vi "Initialize Daemon.vi"(8 "error in":errorcluster, 9 "Data Model":refnum<class "Device Data Model.lvclass">, 11 "Serial Slave in":refnum<class "Serial Slave.lvclass">) -> (0 "error out":errorcluster, 3 "Serial Slave out":refnum<class "Serial Slave.lvclass">)   [LabVIEW 2021, in "Serial Slave.lvclass"]
doc: "This provides an interface for the slave to launch a protocol daemon."
uses:
  Serial Slave.lvclass
  Serial Daemon.vi
  Network Interface/Serial Interface/Serial Shared Components/Serial Shared Components.lvlib
  Transmission Data Unit/Transmission Data Unit.lvclass
  Network Protocol.lvclass
  Transmission Data Unit/Serial Interface/Serial Data Unit.lvclass
  Network Slave.lvclass
  C:/my_projects/projects/Algorithms/Labview/21/Modbus_v121c/Network Protocol/Network Slave/Network Slave.lvclass
  C:/my_projects/projects/Algorithms/Labview/21/Modbus_v121c/Network Protocol/Network Protocol.lvclass
  C:/my_projects/projects/Algorithms/Labview/21/Modbus_v121c/Network Protocol/Network Slave/Serial/Serial Slave.lvclass
  Data Model/Device Data Model.lvclass
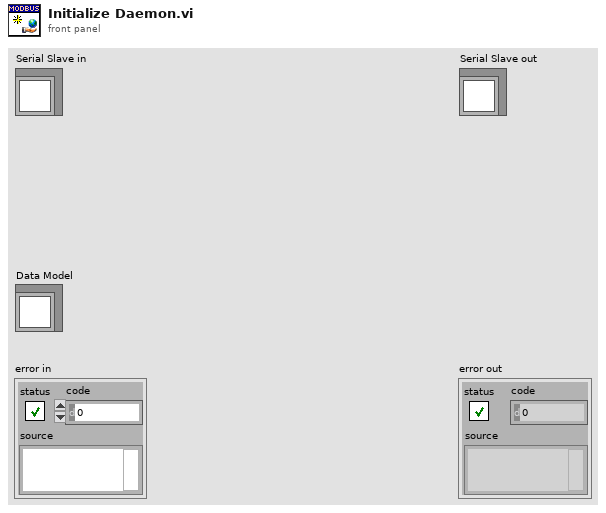
[diagram p1: front panel]
types:
  T1 = enum16{"None", "XON/XOFF", "RTS/CTS", "XON/XOFF & RTS/CTS", "DTR/DSR", "XON/XOFF & DTR/DSR"}
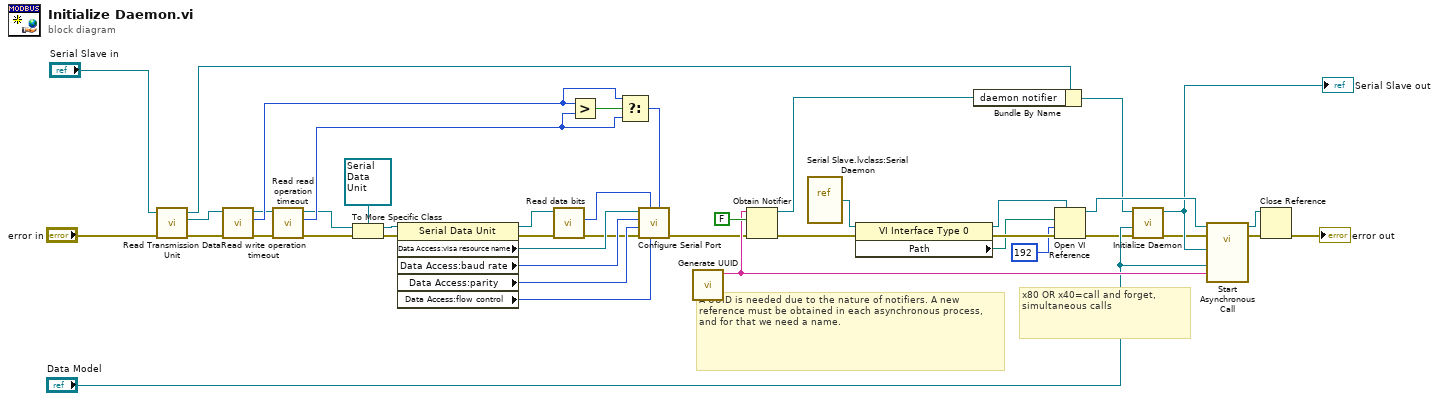
[diagram p0: block diagram]
diagram:
  # "x80 OR x40=call and forget, simultaneous calls"
  # "A UUID is needed due to the nature of notifiers. A new reference must be obtained in each asynchronous process, and for that we need a name."
  n1 = call "Read Transmission Data Unit.vi"("error in (no error)"="error in", "Network Protocol in"="Serial Slave in") -> ("error out"=w13:errorcluster, "Transmission Data Unit"=w5:refnum<class "Transmission Data Unit.lvclass">, "Network Protocol out"=w12:refnum<class "Serial Slave.lvclass">)  [unwired: 7 in]
  n2 = call "Read write operation timeout.vi"("error in (no error)"=w13, "transmission data unit in"=w5) -> ("error out"=w16:errorcluster, "write operation timeout"=w15:i32, "transmission data unit out"=w14:refnum<class "Transmission Data Unit.lvclass">)  [unwired: 7 in]
  n3 = call "Read read operation timeout.vi"("error in (no error)"=w16, "transmission data unit in"=w14) -> ("error out"=w4:errorcluster, "read operation timeout"=w24:i32, "transmission data unit out"=w3:refnum<class "Transmission Data Unit.lvclass">)  [unwired: 7 in]
  n4 = To More Specific Class(target class=refnum<class "Serial Data Unit.lvclass"> refnum ("Serial Data Unit in"), reference=w3, error in=w4) -> (specific class reference=w9:refnum<class "Serial Data Unit.lvclass">, error out=w8:errorcluster)
  n5 = property class="Serial Data Unit"(reference=w9, error in=w8) -> (reference out=w2:refnum<class "Serial Data Unit.lvclass">, error out=w1:errorcluster, "Data Access:visa resource name"=w35:refnum<visa-resource-name>, "Data Access:baud rate"=w33:u32, "Data Access:parity"=w32:enum16{"None", "Odd", "Even", "Mark", "Space"}, "Data Access:flow control"=w31:T1)
  n6 = call-dynamic "Read data bits.vi"("error in (no error)"=w1, "Serial Data Unit in"=w2) -> ("error out"=w7:errorcluster, "data bits"=w34:u16)  [unwired: 7 in, 1 out]
  n7 = Greater?(x=w15, y=w24) -> (0:w25:bool)
  n8 = Select(t=w15, s=w25, f=w24) -> (s? t:f=w23:i32)
  n9 = call "Configure Serial Port.vi"("Timeout"=w23, "Flow Control"=w31, "data bits"=w34, "error in (no error)"=w7, "Parity"=w32, "Baud Rate"=w33, "VISA Refnum in"=w35) -> ("error out"=w30:errorcluster)  [unwired: 4 in]
  n10 = call "Generate UUID.vi"() -> ("UUID"=w37:string)  [unwired: 11 in]
  n11 = Obtain Notifier(name (unnamed)=w37, notification data type=FALSE, error in (no error)=w30) -> (notifier out=w38:refnum<notifier>, error out=w19:errorcluster)  [unwired: 1 in, 1 out]
  n12 = vi-ref "Serial Slave.lvclass:Serial Daemon.vi"() -> (w43:refnum<vi>)
  n13 = property class="VI Interface Type 0"(reference=w43, error in=w19) -> (reference out=w21:refnum<vi>, error out=w42:errorcluster, "Path"=w41:path)
  n14 = Bundle By Name(cluster=w12, "daemon notifier"=w38) -> (w27:refnum<class "Serial Slave.lvclass">)
  n15 = Open VI Reference(type specifier VI Refnum (for type only)=w21, vi path=w41, options=192 ("x .or. y?"), error in (no error)=w42) -> (vi reference=w40:refnum<vi>, error out=w18:errorcluster)  [unwired: 2 in]
  n16 = call-parent "Initialize Daemon.vi"("error in"=w18, "Data Model"="Data Model", "network slave in"=w27) -> ("error out"=w17:errorcluster, "network slave out"=w28:refnum<class "Serial Slave.lvclass">)  [unwired: 7 in]
  "Serial Slave out" <- w28
  n17 = call-by-ref "Start Asynchronous Call"(reference=w40, error in=w17, "UUID"=w37, "Data Model"="Data Model", "serial slave"=w28) -> (reference out=w22:refnum<vi>, error out=w36:errorcluster)  [unwired: 9 in]
  n18 = Close Reference(reference=w22, error in (no error)=w36) -> (error out=→"error out":errorcluster)
